vi "Shift.vi"(8 "error in":errorcluster) -> (0 "error out":errorcluster)   [LabVIEW 2015]
uses:
  Control Button/Save.ctl
  Control Button/Exit.ctl
  <vilib>/addons/database/Connection.llb/DB Tools Open Connec (String).vi
  <vilib>/addons/database/_DB Variant To Data/Database Variant To Data.xnode
  <vilib>/addons/database/NI_Database_API.lvlib
panel:
  in  "Array":T1(array[cluster])
  in  "To-C 2":timestamp=timestamp(3526421399 s since 1904-01-01) format="%<%H:%M:%S\n%d/%m/%Y>T"
  in  "From-C 2":timestamp=timestamp(3526482600 s since 1904-01-01) format="%<%H:%M:%S\n%d/%m/%Y>T"
  out "error out 2":errorcluster
  out "error out":errorcluster
  out "Shift":string="B"
  in  "To-C1":timestamp=timestamp(3526421399 s since 1904-01-01) format="%<%H:%M:%S\n%d/%m/%Y>T"
  in  "From-C1":timestamp=timestamp(3526482600 s since 1904-01-01) format="%<%H:%M:%S\n%d/%m/%Y>T"
  in  "To-B":timestamp=timestamp(3526482599 s since 1904-01-01) format="%<%H:%M:%S\n%d/%m/%Y>T"
  in  "From-B":timestamp=timestamp(3526452000 s since 1904-01-01) format="%<%H:%M:%S\n%d/%m/%Y>T"
  in  "To-A":timestamp=timestamp(3526451999 s since 1904-01-01) format="%<%H:%M:%S\n%d/%m/%Y>T"
  in  "From-A":timestamp=timestamp(3526594200 s since 1904-01-01) format="%<%H:%M:%S\n%d/%m/%Y>T"
  in  "Exit":T2
  in  "Save":T3
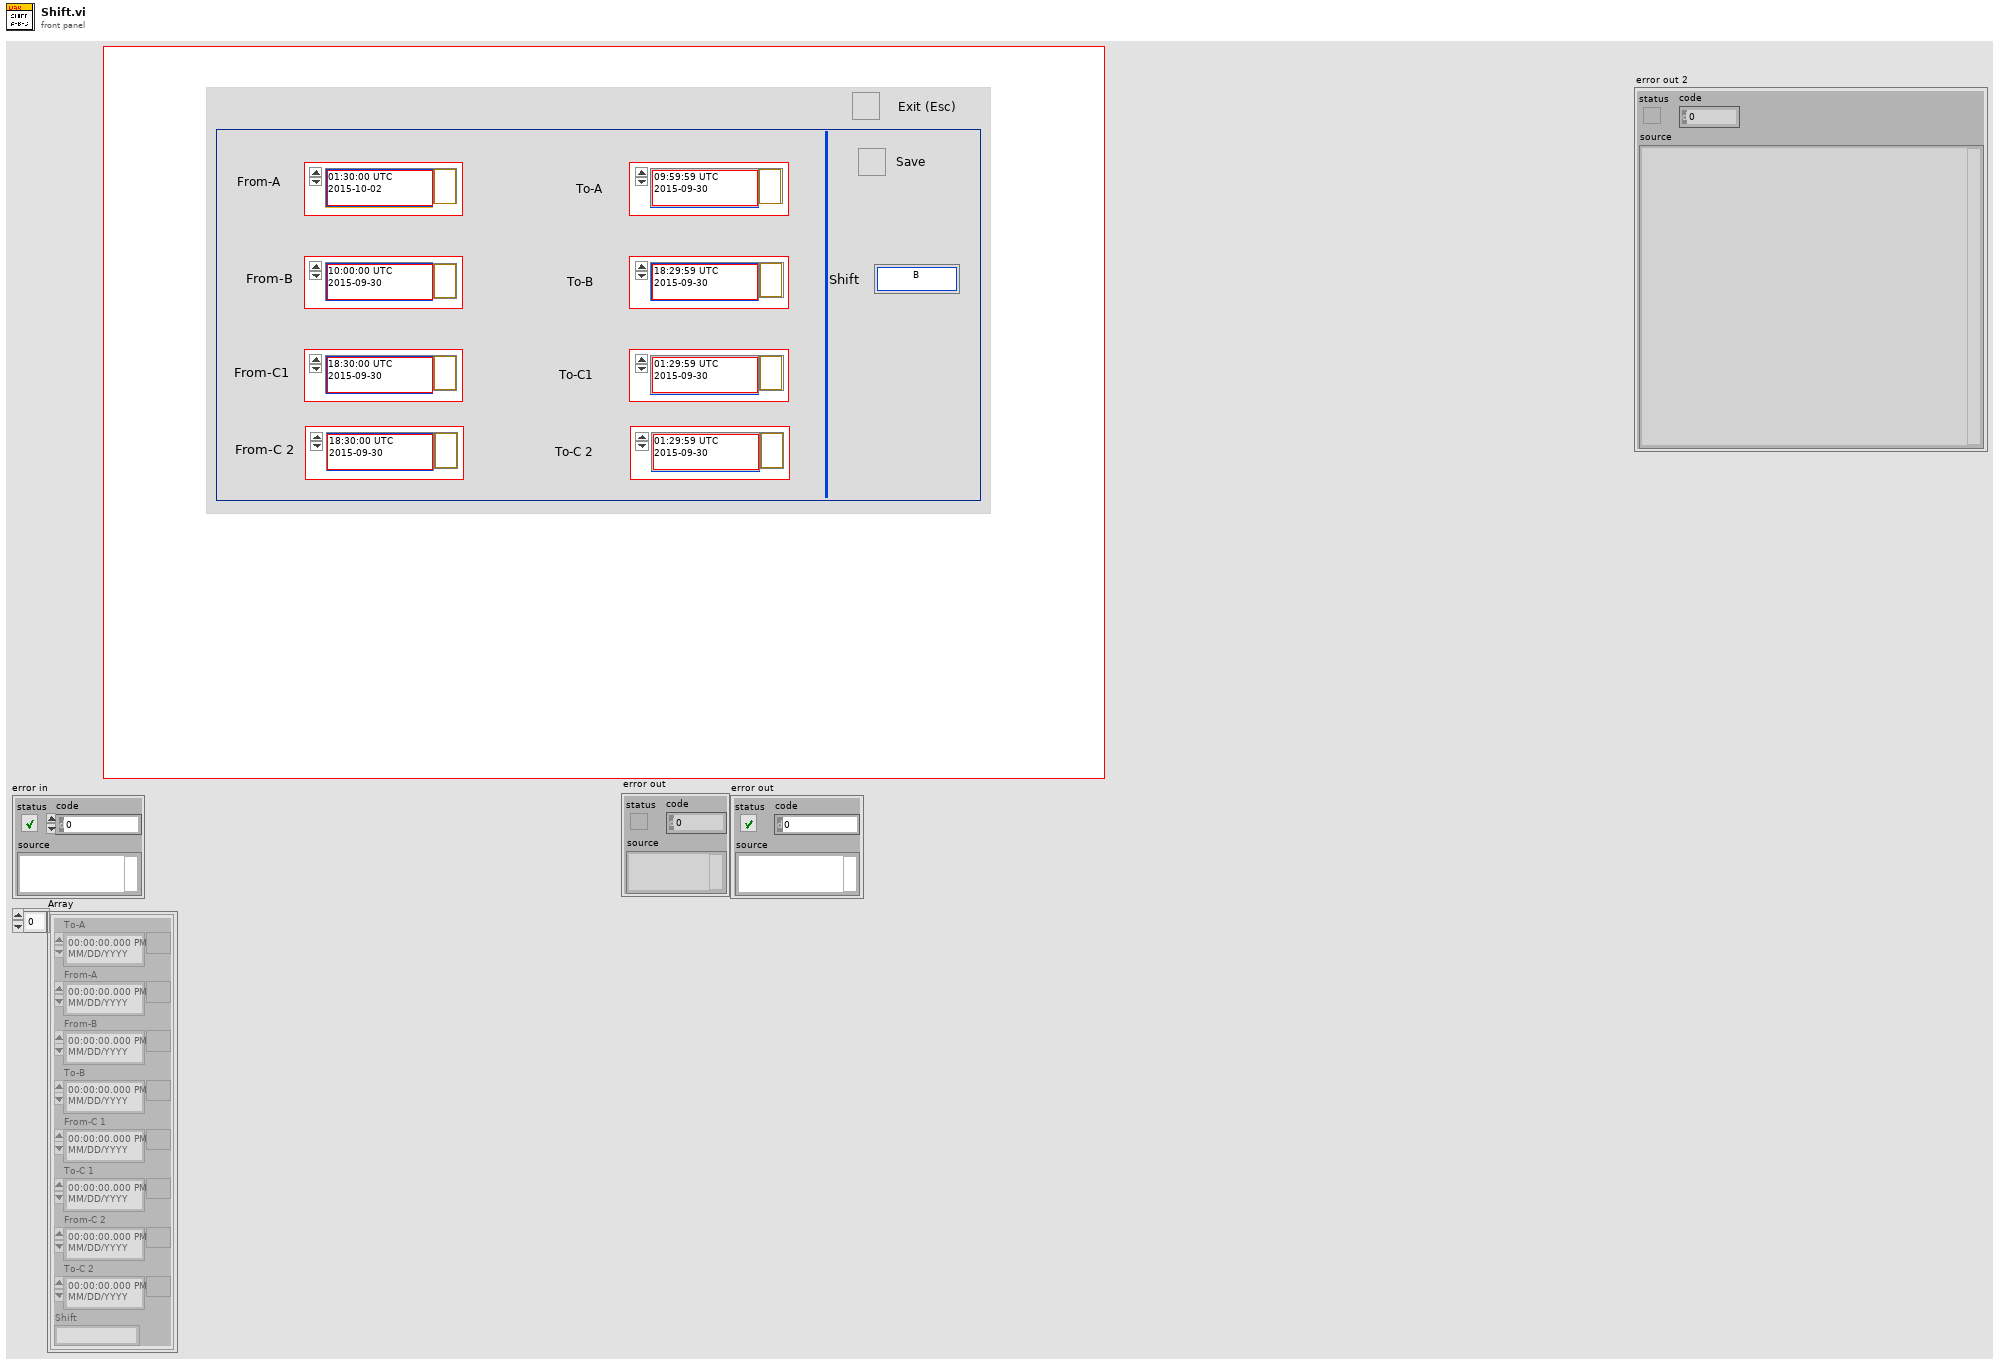
[diagram p1: front panel]
types:
  T1 = cluster{"To-A":timestamp, "From-A":timestamp, "From-B":timestamp, "To-B":timestamp, "From-C 1":timestamp, "To-C 1":timestamp, "From-C 2":timestamp, "To-C 2":timestamp, "Shift":string}[]
  T2 = typedef "Exit.ctl" = bool
  T3 = typedef "Save.ctl" = bool
  T4 = cluster{"To-A":timestamp, "From-A":timestamp, "From-B":timestamp, "To-B":timestamp, "From-C 1":timestamp, "To-C 1":timestamp, "From-C 2":timestamp, "To-C 2":timestamp}
  T5 = cluster{"To-A":timestamp, "From-A":timestamp, "From-B":timestamp, "To-B":timestamp, "From-C 1":timestamp, "To-C 1":timestamp, "From-C 2":timestamp, "To-C 2":timestamp, "Shift":string}
  T6 = typedef "NI_Database_API.lvlib/Conn ObjectReference.ctl" = refnum<k1>
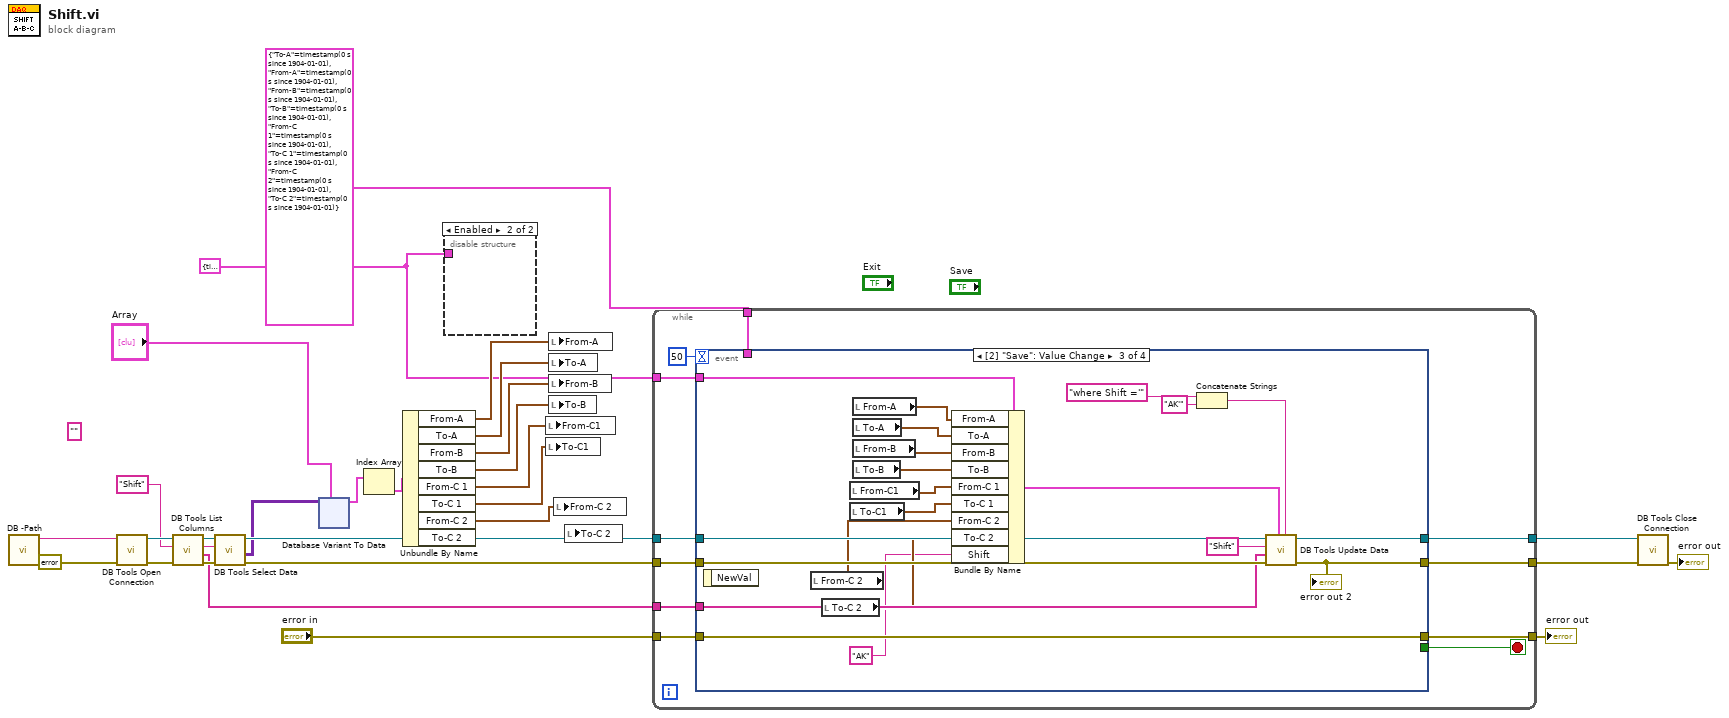
[diagram p0: block diagram]
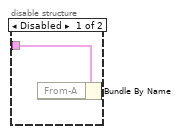
[diagram p2: hidden frame]
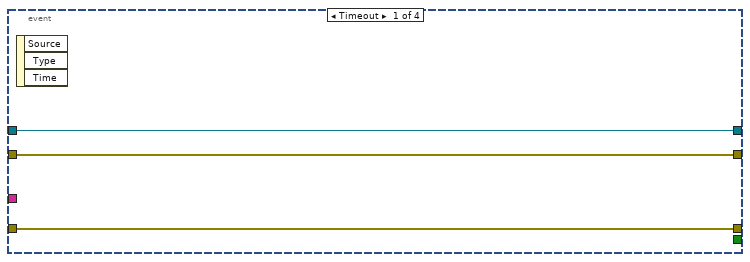
[diagram p3: hidden frame]
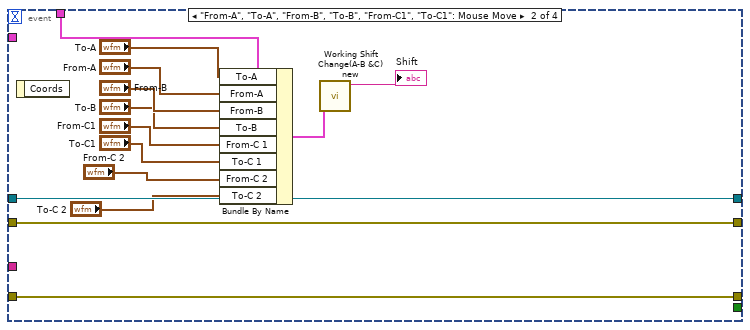
[diagram p4: hidden frame]
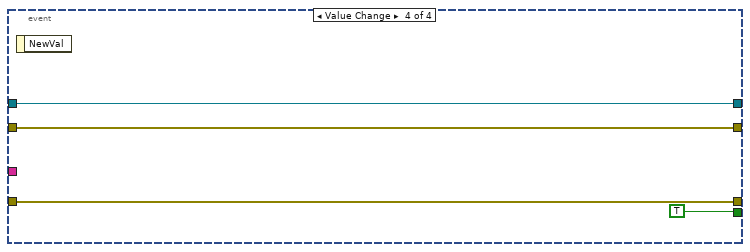
[diagram p5: hidden frame]
diagram:
  (unwired) "" ("Shift")
  w2 = T5 {"To-A"=timestamp(0 s since 1904-01-01), "From-A"=timestamp(0 s since 1904-01-01), "From-B"=timestamp(0 s since 1904-01-01), "To-B"=timestamp(0 s since 1904-01-01), "From-C 1"=timestamp(0 s since 1904-01-01), "To-C 1"=timestamp(0 s since 1904-01-01), "From-C 2"=timestamp(0 s since 1904-01-01), "To-C 2"=timestamp(0 s since 1904-01-01), "Shift"=""} ("Shift")
  w20 = "Shift" ("table")
  n1 = call "DB -Path.vi"() -> ("String"=w29:string)  [unwired: 11 in]
  n2 = call-poly <vilib>:"DB Tools Open Connection.vi"("error in (no error)"=errorcluster {"status"=FALSE, "code"=0, "source"=""}, "connection information"=w29) -> ("error out"=w21:errorcluster, "connection reference"=w22:T6)  [unwired: 6 in]
  n3 = call <vilib>:"DB Tools List Columns.vi"("error in (no error)"=w21, "table"=w20, "connection reference"=w22) -> ("error out"=w18:errorcluster, "columns"=w17:string[], "connection reference out"=w19:T6)  [unwired: 1 in, 1 out]
  n4 = call <vilib>:"DB Tools Select Data.vi"("error in (no error)"=w18, "table"=w20, "connection reference"=w19) -> ("error out"=w27:errorcluster, "data"=w8:variant[][], "connection reference out"=w28:T6)  [unwired: 3 in]
  n5 = xnode "Database Variant To Data"("database variant"=w8, "type"="Array") -> ("data"=w16:T1)  [unwired: 1 in, 1 out]
  n6 = Index Array(array=w16) -> (element=w15:T5)  [unwired: 1 in]
  n7 = Unbundle By Name(w15) -> ("From-A"=w14:timestamp, "To-A"=w13:timestamp, "From-B"=w12:timestamp, "To-B"=w11:timestamp, "From-C 1"=w10:timestamp, "To-C 1"=w9:timestamp, "From-C 2"=w4:timestamp, "To-C 2"=w3:timestamp)
  n8 = disable-structure shown="Enabled" {
    disable-tunnel: w2 -> [w30 _]
    frame Disabled {
      n9 = Bundle By Name(cluster=w30) -> ()  [unwired: 1 in, 1 out]
    }
    frame Enabled {
    }
  }
  n10 = local write "From-C1"(w10) -> ()
  n11 = local write "To-C1"(w9) -> ()
  n12 = local write "From-A"(w14) -> ()
  n13 = local write "To-A"(w13) -> ()
  n14 = local write "From-B"(w12) -> ()
  n15 = local write "To-B"(w11) -> ()
  n16 = local write "From-C 2"(w4) -> ()
  n17 = local write "To-C 2"(w3) -> ()
  n18 = while {
    tunnel: w28 -> [w40]
    tunnel: w27 -> [w39]
    tunnel: [w38] -> w26
    tunnel: [w37] -> w25
    tunnel: w2 -> [w36]
    tunnel: w17 -> [w35]
    tunnel: "error in" -> [w34]
    tunnel: [w33] -> w6
    tunnel: T4 {"To-A"=timestamp(0 s since 1904-01-01), "From-A"=timestamp(0 s since 1904-01-01), "From-B"=timestamp(0 s since 1904-01-01), "To-B"=timestamp(0 s since 1904-01-01), "From-C 1"=timestamp(0 s since 1904-01-01), "To-C 1"=timestamp(0 s since 1904-01-01), "From-C 2"=timestamp(0 s since 1904-01-01), "To-C 2"=timestamp(0 s since 1904-01-01)} ("Shift") -> [w31]
    stop <- w41 stop-if-true
    n19 = event shown="[2] \"Save\": Value Change" {
      selector: _ -> [_ _ _ _]
      dyn-events: _ -> [_ _ _ _]
      timeout: 50 -> [_ _ _ _]
      tunnel: [_ _ _ TRUE] -> w41
      tunnel: w40 -> [w43 w58 w76 w81]
      tunnel: w39 -> [w42 w57 w75 w80]
      tunnel: [w43 w58 w78 w81] -> w38
      tunnel: [w42 w57 w77 w80] -> w37
      tunnel: w36 -> [_ _ w74 _]
      tunnel: w35 -> [_ _ w63 _]
      tunnel: w34 -> [w44 w56 w62 w82]
      tunnel: [w44 w56 w62 w82] -> w33
      tunnel: w31 -> [_ w45 _ _]
      event Timeout {
        n20 = event-data() -> ()  [unwired: 1 in, 3 out]
      }
      event "From-A", "To-A", "From-B", "To-B", "From-C1", "To-C1": Mouse Move {
        n21 = event-data() -> ()  [unwired: 1 in, 1 out]
        n22 = Bundle By Name(cluster=w45, "To-A"="To-A", "From-A"="From-A", "From-B"="From-B", "To-B"="To-B", "From-C 1"="From-C1", "To-C 1"="To-C1", "From-C 2"="From-C 2", "To-C 2"="To-C 2") -> (w46:T4)
        n23 = call "Working Shift Change(A-B &C) new.vi"("input cluster"=w46) -> ("Shift Change"=→"Shift":string)  [unwired: 10 in]
      }
      event Value Change {
        n24 = event-data() -> ()  [unwired: 1 in, 1 out]
        n25 = local read "From-C 2"() -> (w61:timestamp)
        n26 = local read "To-C 2"() -> (w60:timestamp)
        n27 = local read "From-C1"() -> (w69:timestamp)
        n28 = local read "To-C1"() -> (w68:timestamp)
        n29 = local read "From-A"() -> (w73:timestamp)
        n30 = local read "To-A"() -> (w72:timestamp)
        n31 = local read "From-B"() -> (w71:timestamp)
        n32 = local read "To-B"() -> (w70:timestamp)
        n33 = Bundle By Name(cluster=w74, "From-A"=w73, "To-A"=w72, "From-B"=w71, "To-B"=w70, "From-C 1"=w69, "To-C 1"=w68, "From-C 2"=w61, "To-C 2"=w60, "Shift"="AK") -> (w79:T5)
        n34 = Concatenate Strings("where Shift ='" ("string"), "AK'" ("string")) -> (w64:string)
        n35 = call <vilib>:"DB Tools Update Data.vi"("condition"=w64, "data"=w79, "error in (no error)"=w75, "columns"=w63, "table"="Shift", "connection reference"=w76) -> ("error out"=w77:errorcluster, "connection reference out"=w78:T6)  [unwired: 4 in]
        "error out 2" <- w77
      }
      event Value Change {
        n36 = event-data() -> ()  [unwired: 1 in, 1 out]
      }
    }
  }
  "error out" <- w6
  n37 = call <vilib>:"DB Tools Close Connection.vi"("error in (no error)"=w25, "connection reference"=w26) -> ("error out"=→"error out":errorcluster)  [unwired: 5 in]
